vi "MQTT_Client.vi"(7 "JPG":refnum<vi>, 10 "queueName":string="PV_script", 11 "Console Reference":refnum<vi>) -> ()   [LabVIEW 2022 SP3]
panel:
  in  "Tab Control":enum32{"Connect", "connected"}(tab)=enum."connected"
  in  "Connect":bool
  out "success?":bool
  out "Connection":string
  in  "add sub":bool
  in  "clear buffer":bool
  in  "pub":bool
  in  "Publish message":string="Hello"
  in  "Publish topic":string="test"
  out "Buffer":i32(slide)=14 scale=0.0..100.0
  in  "read":bool
  out "buffer":string
  in  "subscribe topics":string[](array[string])=["angles", "test"]
  in  "Broker Address":string="127.0.0.1"
  in  "Client ID":string="LabVIEW"
  # "Note this only works if you are running Python with paho installed"
  # "MQTT"
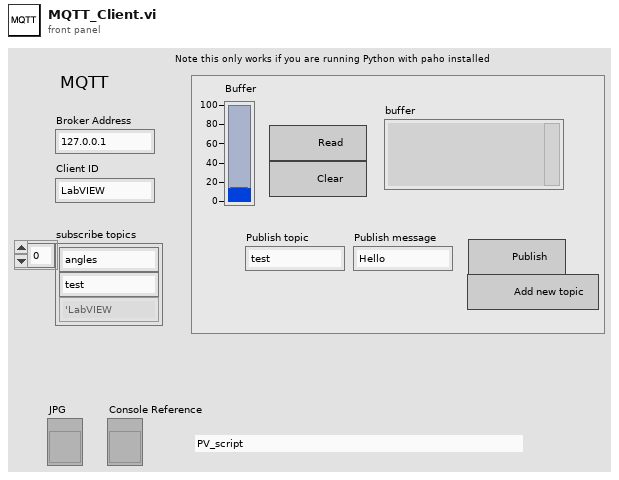
[diagram p1: front panel]
types:
  T1 = typedef "Preferences.ctl" = cluster{"python":string, "arduino CLI":path, "pythonCodes":cluster{"pythonCode":path, "Color":u32}[], "FontSize":u8, "Text Colors":cluster{"Quote":u32, "function":u32, "Python":u32, "Comment":u32, "Triple Quote":u32, "Text":u32}, "SSH Logins":cluster{"IP Address":string, "Username":string, "password":string}[], "packet size":u8}
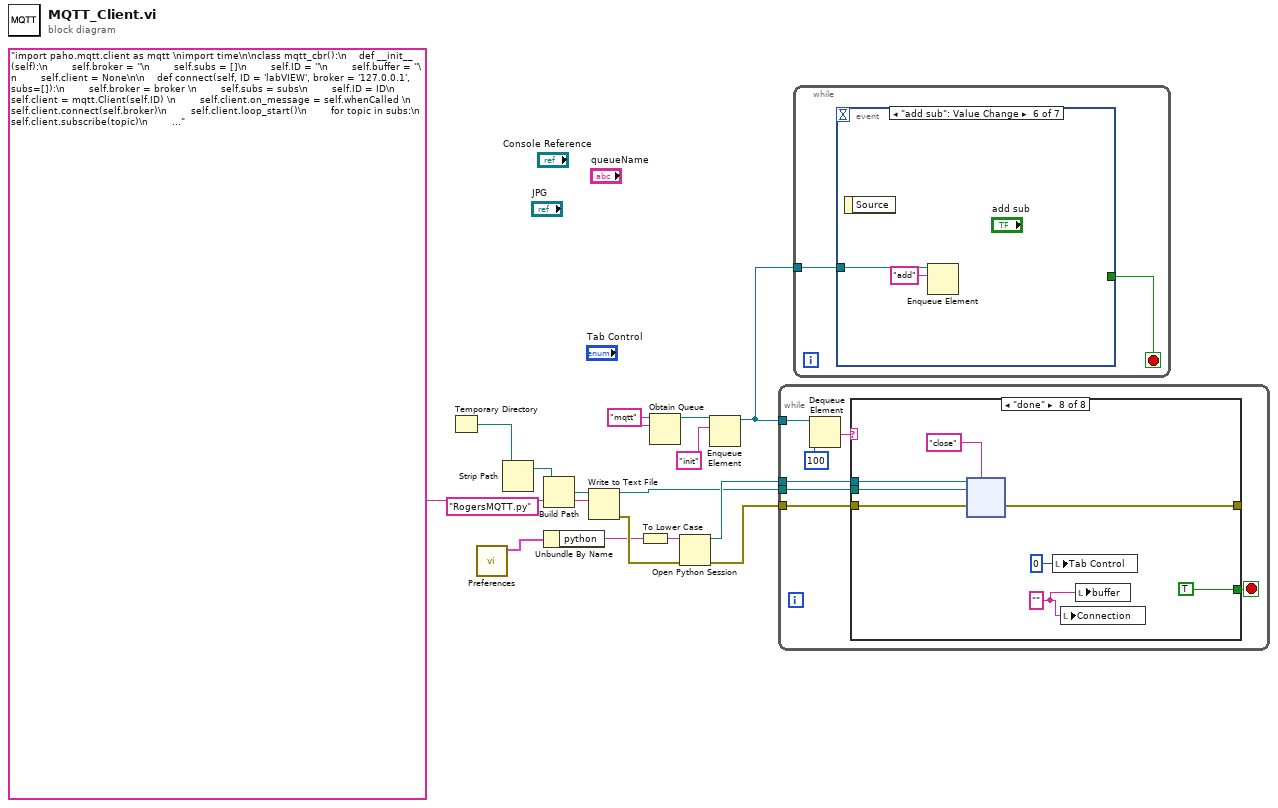
[diagram p0: block diagram]
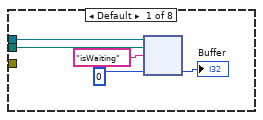
[diagram p2: hidden frame]
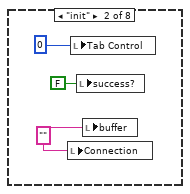
[diagram p3: hidden frame]
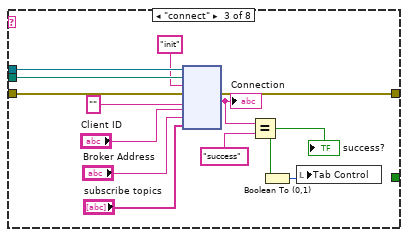
[diagram p4: hidden frame]
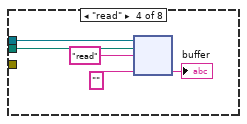
[diagram p5: hidden frame]
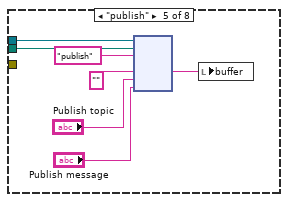
[diagram p6: hidden frame]
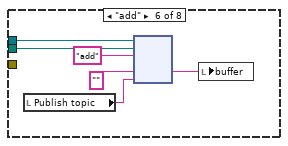
[diagram p7: hidden frame]
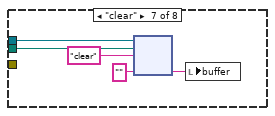
[diagram p8: hidden frame]
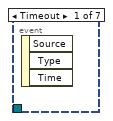
[diagram p9: hidden frame]
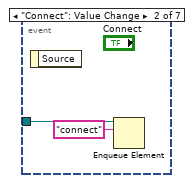
[diagram p10: hidden frame]
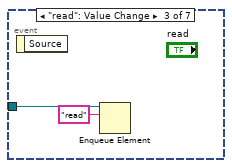
[diagram p11: hidden frame]
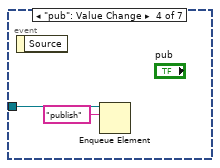
[diagram p12: hidden frame]
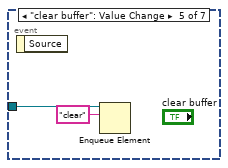
[diagram p13: hidden frame]
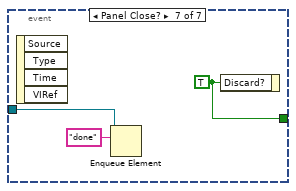
[diagram p14: hidden frame]
diagram:
  w9 = "mqtt" ("name (unnamed)")
  n1 = Temporary Directory() -> (w10:path)
  n2 = call "Preferences.vi"() -> ("Preferences out"=w2:T1)  [unwired: 10 in, 1 out]
  n3 = Strip Path(path=w10) -> (stripped path=w15:path)  [unwired: 1 out]
  n4 = Build Path(base path=w15, name or relative path="RogersMQTT.py") -> (appended path=w7:path)
  n5 = Unbundle By Name(w2) -> ("python"=w1:string)
  n6 = Write to Text File(file (use dialog)=w7, text="import paho.mqtt.client as mqtt \nimport time\n\nclass mqtt_cbr():\n    def __init__(self):\n        self.broker = ''\n        self.subs = []\n        self.ID = ''\n        self.buffer = ''\n        self.client = None\n\n    def connect(self, ID = 'labVIEW', broker = '127.0.0.1', subs=[]):\n        self.broker = broker \n        self.subs = subs\n        self.ID = ID\n        self.client = mqtt.Client(self.ID) \n        self.client.on_message = self.whenCalled \n        self.client.connect(self.broker)\n        self.client.loop_start()\n        for topic in subs:\n            self.client.subscribe(topic)\n        \n    def add_sub(self, topic):\n        '''add a subscriber - pass in the topic name in quotes'''\n        self.subs.append(topic)\n        if self.client:\n            self.client.subscribe(topic)\n        \n    def whenCalled(self, client, userdata, message):\n        '''callback for new message'''\n        self.buffer += message.payload.decode(\"utf-8\")\n        \n    def publish(self, topic, message):\n        '''publish to a topic - pass in the topic name and message in quotes '''\n        self.client.publish(topic, message)\n        \n    def read(self):\n        '''return buffer contents (without erasing)'''\n        return self.buffer\n        \n    def isWaiting(self):\n        '''return the size of the buffer'''\n        return len(self.buffer)\n\n    def clearBuffer(self):\n        '''erase everything in the buffer'''\n        self.buffer = ''\n        \n    def close(self):\n        '''close the connection'''\n        if self.client:\n            self.client.loop_stop()  # close any old connection\n\nclient = mqtt_cbr()\n\ndef init(ID = 'labVIEW', broker = '127.0.0.1', subs=[]):\n    try:\n        client.connect(ID,broker,subs)\n        return 'success'\n    except Exception as e:\n        return str(e)\n    \ndef add(topic):\n    try:\n        client.add_sub(topic)\n        return 'success'\n    except Exception as e:\n        return str(e)\n\ndef read():\n    try:\n        return client.read()\n    except Exception as e:\n        return str(e)\n\ndef isWaiting():\n    try:\n        return client.isWaiting()\n    except:\n        return -1\n\ndef clear():\n    try:\n        client.clearBuffer()\n        return 'success'\n    except Exception as e:\n        return str(e)\n\ndef publish(topic, msg):\n    try:\n        client.publish(topic, msg)\n        return 'success'\n    except Exception as e:\n        return str(e)\n\ndef close():\n    return client.close()\n\n") -> (error out=w14:errorcluster)  [unwired: 2 in, 2 out]
  n7 = To Lower Case(string=w1) -> (all lower case string=w13:string)
  n8 = Obtain Queue(name (unnamed)=w9, element data type=w9) -> (queue out=w4:refnum<queue>)  [unwired: 3 in, 2 out]
  n9 = Open Python Session(python version=w13, 3:w14) -> (session out=w8:refnum<k35>, error out=w6:errorcluster)  [unwired: 1 in]
  n10 = Enqueue Element(queue=w4, element="init") -> (queue out=w3:refnum<queue>)  [unwired: 2 in, 2 out]
  n11 = while {
    tunnel: w3 -> [w22]
    tunnel: w8 -> [w20]
    tunnel: w7 -> [w19]
    tunnel: w6 -> [w18]
    stop <- w17 stop-if-true
    n12 = Dequeue Element(queue=w22, timeout in ms (-1)=100) -> (element=w21:string)  [unwired: 1 in, 3 out]
    n13 = case shown="\"done\"" w21 {
      tunnel: w20 -> [w25 _ w40 w46 w54 w60 w65 w72]
      tunnel: w19 -> [w24 _ w39 w45 w53 w59 w64 w71]
      tunnel: w18 -> [_ _ w37 _ _ _ _ w70]
      tunnel: [_ _ _ _ _ _ _ TRUE] -> w17
      tunnel: [_ _ w31 _ _ _ _ w69] -> _
      frame Default {
        n14 = node(w25, w24, "isWaiting" ("function name"), 0) -> (→"Buffer":i32)  [unwired: 1 in, 4 out]
      }
      frame "init" {
        w28 = "" ("name or relative path")
        n15 = local write "Connection"(w28) -> ()
        n16 = local write "Tab Control"(0 ("timeout in ms (-1)")) -> ()
        n17 = local write "success?"(FALSE ("success?")) -> ()
        n18 = local write "buffer"(w28) -> ()
      }
      frame "connect" {
        n19 = node(w40, w39, "init" ("function name"), w37, "" ("function name"), "Client ID", "Broker Address", "subscribe topics") -> (w31:errorcluster, w34:string)  [unwired: 3 in, 3 out]
        "Connection" <- w34
        n20 = Equal?(x=w34, y="success" ("function name")) -> (x = y?=w33:bool)
        "success?" <- w33
        n21 = Boolean To (0,1)(Boolean=w33) -> (0, 1=w32:i16)
        n22 = local write "Tab Control"(w32) -> ()
      }
      frame "read" {
        n23 = node(w46, w45, "read" ("function name"), "" ("function name")) -> (→"buffer":string)  [unwired: 1 in, 4 out]
      }
      frame "publish" {
        n24 = node(w54, w53, "publish" ("function name"), "" ("function name"), "Publish topic", "Publish message") -> (w49:string)  [unwired: 3 in, 4 out]
        n25 = local write "buffer"(w49) -> ()
      }
      frame "add" {
        n26 = local read "Publish topic"() -> (w56:string)
        n27 = node(w60, w59, "add" ("function name"), "" ("function name"), w56) -> (w57:string)  [unwired: 2 in, 4 out]
        n28 = local write "buffer"(w57) -> ()
      }
      frame "clear" {
        n29 = node(w65, w64, "clear" ("function name"), "" ("function name")) -> (w62:string)  [unwired: 1 in, 4 out]
        n30 = local write "buffer"(w62) -> ()
      }
      frame "done" {
        w67 = "" ("name or relative path")
        n31 = node(w72, w71, "close" ("function name"), w70) -> (w69:errorcluster)  [unwired: 2 in, 3 out]
        n32 = local write "Tab Control"(0 ("timeout in ms (-1)")) -> ()
        n33 = local write "Connection"(w67) -> ()
        n34 = local write "buffer"(w67) -> ()
      }
    }
  }
  n35 = while {
    tunnel: w3 -> [w76]
    stop <- w75 stop-if-true
    n36 = event shown="[5] \"add sub\": Value Change" {
      selector: _ -> [_ _ _ _ _ _ _]
      dyn-events: _ -> [_ _ _ _ _ _ _]
      timeout: _ -> [_ _ _ _ _ _ _]
      tunnel: w76 -> [_ w78 w80 w82 w84 w86 w87]
      tunnel: [_ _ _ _ _ _ w89] -> w75
      event Timeout {
        n37 = event-data() -> ()  [unwired: 1 in, 3 out]
      }
      event "Connect": Value Change {
        n38 = event-data() -> ()  [unwired: 1 in, 1 out]
        n39 = Enqueue Element(queue=w78, element="connect") -> ()  [unwired: 2 in, 3 out]
      }
      event "read": Value Change {
        n40 = event-data() -> ()  [unwired: 1 in, 1 out]
        n41 = Enqueue Element(queue=w80, element="read") -> ()  [unwired: 2 in, 3 out]
      }
      event "pub": Value Change {
        n42 = event-data() -> ()  [unwired: 1 in, 1 out]
        n43 = Enqueue Element(queue=w82, element="publish") -> ()  [unwired: 2 in, 3 out]
      }
      event "clear buffer": Value Change {
        n44 = event-data() -> ()  [unwired: 1 in, 1 out]
        n45 = Enqueue Element(queue=w84, element="clear") -> ()  [unwired: 2 in, 3 out]
      }
      event "add sub": Value Change {
        n46 = event-data() -> ()  [unwired: 1 in, 1 out]
        n47 = Enqueue Element(queue=w86, element="add") -> ()  [unwired: 2 in, 3 out]
      }
      event Panel Close? {
        w89 = TRUE ("Discard?")
        n48 = event-data() -> ()  [unwired: 1 in, 4 out]
        n49 = Enqueue Element(queue=w87, element="done") -> ()  [unwired: 2 in, 3 out]
        n50 = event-data("Discard?"=w89) -> ()  [unwired: 1 in, 1 out]
      }
    }
  }
